vi "Img2TFMatrix_001.vi"() -> ()   [LabVIEW 2018]
panel:
  out "subarray":bool[](array[boolean])
  in  "stop":bool
  in  "index (row)":i32
  out "1-bit pixmap":bool[][](array[boolean])
  in  "Path":path
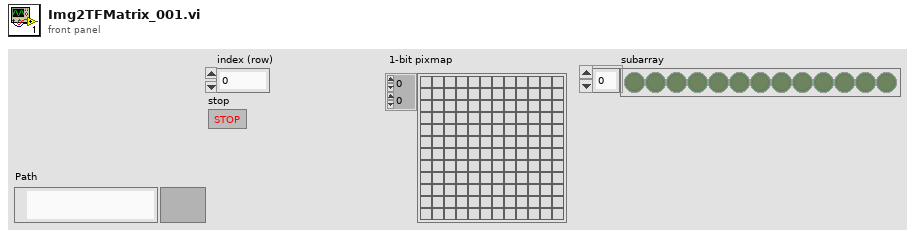
[diagram p1: front panel]
types:
  T1 = typedef "imagedata.ctl" = cluster{"image type":i32, "image depth":i32, "image":u8[], "mask":u8[], "colors":u32[], "Rectangle":cluster{"left":i16, "top":i16, "right":i16, "bottom":i16}}
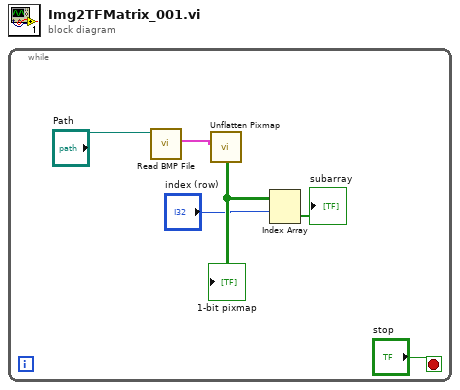
[diagram p0: block diagram]
diagram:
  n1 = while {
    stop <- "stop" stop-if-true
    n2 = call <vilib>:"Read BMP File.vi"("path to BMP file"="Path") -> ("image data"=w5:T1)  [unwired: 8 in, 2 out]
    n3 = call <vilib>:"Unflatten Pixmap.vi"("image data"=w5) -> ("1-bit pixmap"=w4:bool[][])  [unwired: 4 in, 6 out]
    "1-bit pixmap" <- w4
    n4 = Index Array(array=w4, index (row)="index (row)") -> (element=→"subarray":bool[])  [unwired: 1 in]
  }
